vi "Queue - Enqueue.vi"(6 "Priority Message? (F)":bool, 8 "error in (no error)":errorcluster, 9 "Message Data":variant, 10 "Message":string, 11 "Message Queue":refnum<queue>) -> (0 "error out":errorcluster, 3 "dup Message Queue":refnum<queue>)   [LabVIEW 2024, in "QMH Messaging.lvlib"]
uses:
  QMH Messaging.lvlib
  General Type Defs/Queue Message.ctl
  General Type Defs/General Type Defs.lvlib
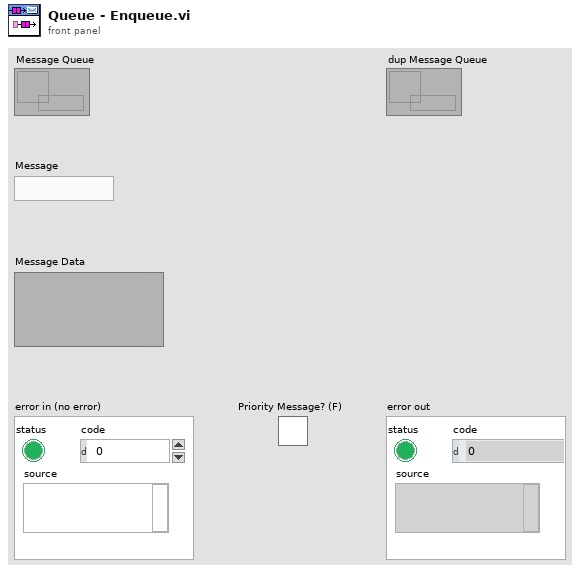
[diagram p1: front panel]
types:
  T1 = typedef "General Type Defs.lvlib/Queue Message.ctl" = cluster{"Message":string, "Value":variant}
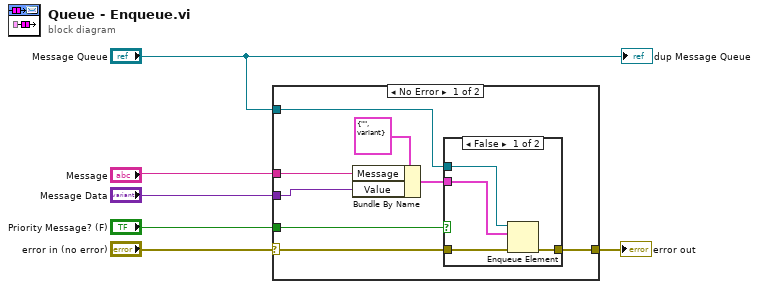
[diagram p0: block diagram]
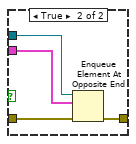
[diagram p2: hidden frame]
diagram:
  n1 = case shown="No Error" "error in (no error)" {
    selector: "error in (no error)" -> [w7 w23]
    tunnel: "Message Queue" -> [w13 _]
    tunnel: [w12 w23] -> w5
    tunnel: "Priority Message? (F)" -> [w11 _]
    tunnel: "Message Data" -> [w10 _]
    tunnel: "Message" -> [w9 _]
    frame No Error {
      n2 = Bundle By Name(cluster=T1 {"Message"="", "Value"=variant} ("Queue Message"), "Message"=w9, "Value"=w10) -> (w14:T1)
      n3 = case shown="False" w11 {
        tunnel: w7 -> [w18 w22]
        tunnel: [w17 w21] -> w12
        tunnel: w13 -> [w16 w20]
        tunnel: w14 -> [w15 w19]
        frame False {
          n4 = Enqueue Element(queue=w16, element=w15, error in (no error)=w18) -> (error out=w17:errorcluster)  [unwired: 1 in, 2 out]
        }
        frame True {
          n5 = Enqueue Element At Opposite End(queue=w20, element=w19, error in (no error)=w22) -> (error out=w21:errorcluster)  [unwired: 1 in, 2 out]
        }
      }
    }
    frame Error {
    }
  }
  "error out" <- w5
  "dup Message Queue" <- "Message Queue"
